vi "Simulated data.vi"(8 "error in":errorcluster, 11 "run/reset":bool=TRUE) -> (0 "error out":errorcluster, 3 "Array":u8[](array[numeric]))   [LabVIEW 2014]
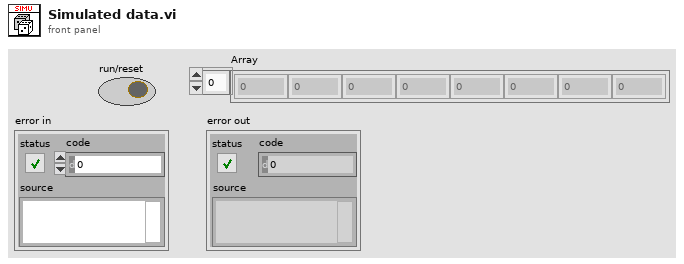
[diagram p1: front panel]
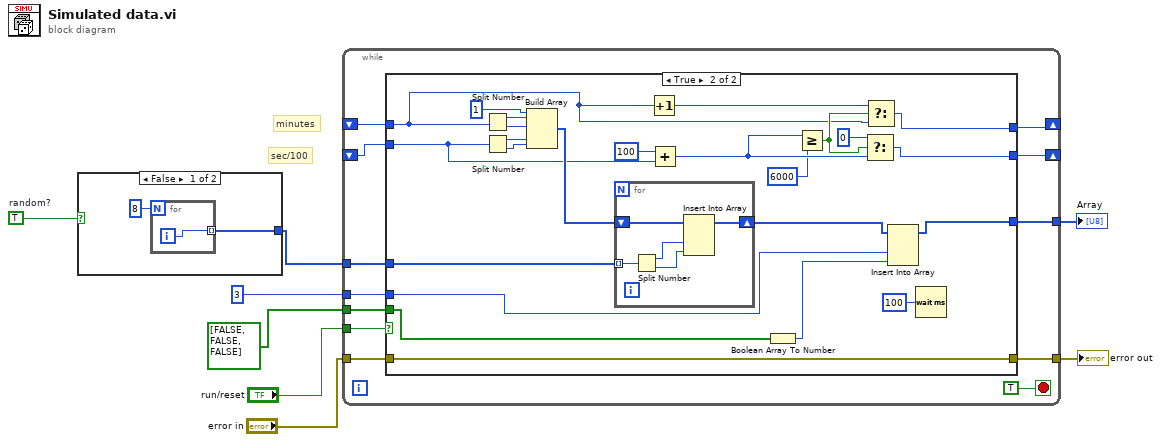
[diagram p0: block diagram]
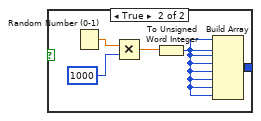
[diagram p2: hidden frame]
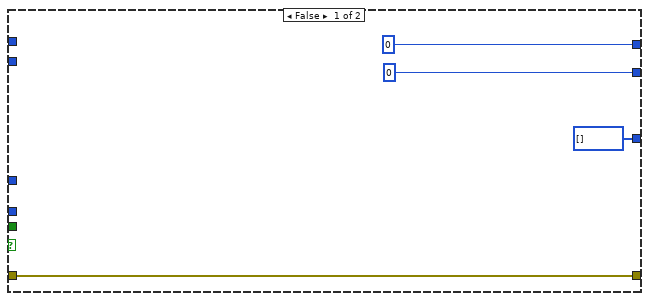
[diagram p3: hidden frame]
diagram:
  w1 = TRUE  # random?
  # "sec/100"
  # "minutes"
  n1 = case shown="False" w1 {
    tunnel: [w10 w16] -> w2
    frame False {
      n2 = for {
        N: 8 -> [_]
        tunnel: [w11] -> w10 mode=indexing
        i -> [w11]
      }
    }
    frame True {
      n3 = Random Number (0-1)() -> (number: 0 to 1=w15:dbl)
      n4 = Multiply(x=w15, y=u16 1000) -> (x*y=w13:dbl)
      n5 = To Unsigned Word Integer(number=w13) -> (unsigned 16bit integer=w12:u16)
      n6 = Build Array(w12, w12, w12, w12, w12, w12, w12, w12) -> (w16:u16[])
    }
  }
  n7 = while {
    shift-right: [w25] -> _
    shift-left: _ -> [w24]
    tunnel: w2 -> [w27]
    tunnel: "run/reset" -> [w26]
    tunnel: "error in" -> [w23]
    tunnel: [w22] -> w6
    tunnel: 3 -> [w21]
    tunnel: bool[] [FALSE, FALSE, FALSE] ("Boolean array") -> [w20]
    tunnel: [w19] -> w3
    shift-right: [w18] -> _
    shift-left: _ -> [w17]
    stop <- TRUE stop-if-true
    n8 = case shown="True" w26 {
      tunnel: w27 -> [_ w56]
      tunnel: [u16 0 w38] -> w25
      tunnel: w24 -> [_ w36]
      tunnel: w23 -> [w31 w50]
      tunnel: [w31 w50] -> w22
      tunnel: w21 -> [_ w47]
      tunnel: w20 -> [_ w48]
      tunnel: [u16[] [] w44] -> w19
      tunnel: [u16 0 w39] -> w18
      tunnel: w17 -> [_ w43]
      frame False {
      }
      frame True {
        n9 = Split Number(x=w36) -> (hi(x)=w55:u8, lo(x)=w54:u8)
        n10 = Split Number(x=w43) -> (hi(x)=w53:u8, lo(x)=w52:u8)
        n11 = Build Array(u8 1 ("element"), w55, w54, w53, w52) -> (w49:u8[])
        n12 = for {
          tunnel: w56 -> [w57] mode=indexing
          shift-right: [w58] -> w45
          shift-left: w49 -> [w61]
          n13 = Split Number(x=w57) -> (hi(x)=w60:u16, lo(x)=w59:u16)
          n14 = Insert Into Array(array=w61, new element #1=w60, new element #2=w59) -> (w58:u8[])  [unwired: 1 in]
        }
        n15 = Increment(x=w36) -> (x+1=w35:u16)
        n16 = Add(x=u16 100, y=w43) -> (x+y=w41:u16)
        n17 = Boolean Array To Number(Boolean array=w48) -> (number=w46:u32)
        n18 = Greater Or Equal?(x=w41, y=u16 6000 ("x")) -> (x >= y?=w37:bool)
        n19 = Select(t=u16 0, s=w37, f=w41) -> (s? t:f=w39:u16)
        n20 = Select(t=w35, s=w37, f=w36) -> (s? t:f=w38:u16)
        n21 = Insert Into Array(array=w45, new element #1=w47, new element #2=w46) -> (w44:u8[])  [unwired: 1 in]
        n22 = Wait (ms)(milliseconds to wait=u32 100) -> ()  [unwired: 1 out]
      }
    }
  }
  "error out" <- w6
  "Array" <- w3
